vi "MODbus_TRANSMITTER_EXAMPLE.vi"() -> ()   [LabVIEW 2014]
panel:
  out "SUCESS":bool
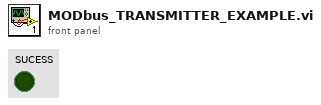
[diagram p1: front panel]
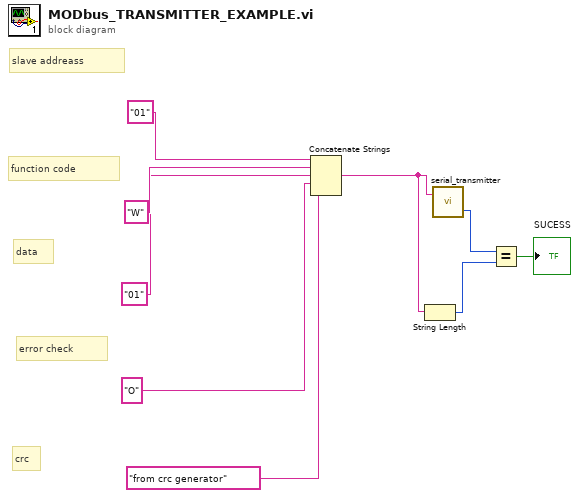
[diagram p0: block diagram]
diagram:
  # "crc"
  # "error check"
  # "data"
  # "function code"
  # "slave addreass"
  n1 = Concatenate Strings("01", "W", "01", "O", "from crc generator") -> (w4:string)
  n2 = String Length(string=w4) -> (length=w3:i32)
  n3 = call "serial_transmitter.vi"("write buffer"=w4) -> ("return count"=w5:u32)  [unwired: 1 in, 1 out]
  n4 = Equal?(x=w5, y=w3) -> (x = y?=→"SUCESS":bool)
